vi "Write Test Result.vi"(9 "Position":u32, 10 "Test Passed":bool, 11 "Test Class.lvclass":refnum<class "Test Class.lvclass">) -> ()   [LabVIEW 2015]
uses:
  Classes/Application/Class/Application.lvclass
  Test Class.lvclass
  <vilib>/Cree, Inc/Cree Test Framework/Core Launcher/Core Launcher.lvlib
  <vilib>/Cree, Inc/Cree Test Framework/Core Launcher/Core Manager Methods -- Enum.ctl
  <vilib>/Cree, Inc/Cree Test Framework/Classes/Data/Data Repo/Class/Data Repo.lvclass
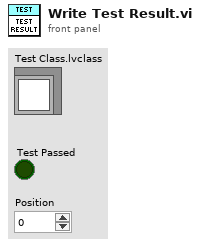
[diagram p1: front panel]
types:
  T1 = typedef "Core Launcher.lvlib/Core Manager Methods -- Enum.ctl" = enum16{"Spawn Objects", "Get Objects", "Destroy Objects"}
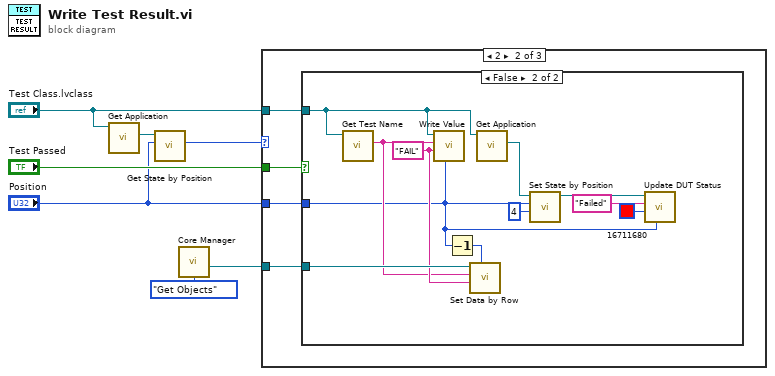
[diagram p0: block diagram]
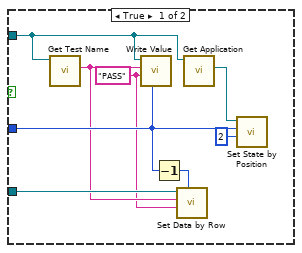
[diagram p3: hidden frame]
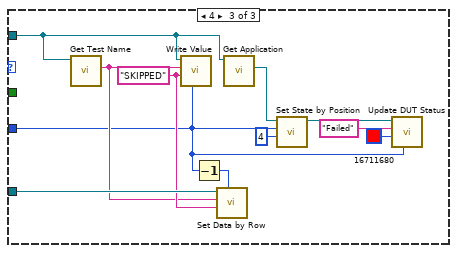
[diagram p4: hidden frame]
diagram:
  n1 = call "Get Application.vi"("Test Class in"="Test Class.lvclass") -> ("Application.lvlib:Application.lvclass"=w6:refnum<class "Application.lvclass">)  [unwired: 9 in, 1 out]
  n2 = call-dynamic "Get State by Position.vi"("Position"="Position", "Application in"=w6) -> ("State"=w4:u32)  [unwired: 7 in, 2 out]
  n3 = call <vilib>:"Core Manager.vi"("Method"=Core_Manager_Methods_--_Enum."Get Objects") -> ("Data Repo"=w2:refnum<class "Data Repo.lvclass">)  [unwired: 6 in, 4 out]
  n4 = case shown="2" w4 {
    tunnel: "Test Passed" -> [_ w11 _]
    tunnel: "Position" -> [_ w10 w31]
    tunnel: "Test Class.lvclass" -> [_ w9 w32]
    tunnel: w2 -> [_ w8 w41]
    frame Default {
    }
    frame 2 {
      n5 = case shown="False" w11 {
        tunnel: w10 -> [w16 w20]
        tunnel: w9 -> [w12 w21]
        tunnel: w8 -> [w17 w25]
        frame True {
          w13 = "PASS" ("Message")
          n6 = call "Get Test Name.vi"("Test Class in"=w12) -> ("Test Name"=w14:string)  [unwired: 9 in, 1 out]
          n7 = call "Write Value.vi"("Position"=w16, "Value"=w13, "Label"=w14, "Test Class in"=w12) -> ()  [unwired: 7 in, 1 out]
          n8 = Decrement(x=w16) -> (x-1=w15:u32)
          n9 = call <vilib>:"Set Data by Row.vi"("Row"=w15, "Value"=w13, "Header"=w14, "Acrobat Template in"=w17) -> ()  [unwired: 6 in, 2 out]
          n10 = call "Get Application.vi"("Test Class in"=w12) -> ("Application.lvlib:Application.lvclass"=w19:refnum<class "Application.lvclass">)  [unwired: 9 in, 1 out]
          n11 = call-dynamic "Set State by Position.vi"("State"=u32 2, "Position"=w16, "Application in"=w19) -> ()  [unwired: 7 in, 2 out]
        }
        frame False {
          w23 = "FAIL" ("Message")
          n12 = call "Get Test Name.vi"("Test Class in"=w21) -> ("Test Name"=w22:string)  [unwired: 9 in, 1 out]
          n13 = call "Write Value.vi"("Position"=w20, "Value"=w23, "Label"=w22, "Test Class in"=w21) -> ()  [unwired: 7 in, 1 out]
          n14 = Decrement(x=w20) -> (x-1=w24:u32)
          n15 = call <vilib>:"Set Data by Row.vi"("Row"=w24, "Value"=w23, "Header"=w22, "Acrobat Template in"=w25) -> ()  [unwired: 6 in, 2 out]
          n16 = call "Get Application.vi"("Test Class in"=w21) -> ("Application.lvlib:Application.lvclass"=w30:refnum<class "Application.lvclass">)  [unwired: 9 in, 1 out]
          n17 = call-dynamic "Set State by Position.vi"("State"=u32 4, "Position"=w20, "Application in"=w30) -> ("Application out"=w28:refnum<class "Application.lvclass">)  [unwired: 7 in, 1 out]
          n18 = call "Update DUT Status.vi"("Position"=w20, "BG Color"=u32 16711680, "Message ('')"="Failed", "Application in"=w28) -> ()  [unwired: 6 in, 2 out]
        }
      }
    }
    frame 4 {
      w34 = "SKIPPED" ("Message")
      n19 = call "Get Test Name.vi"("Test Class in"=w32) -> ("Test Name"=w33:string)  [unwired: 9 in, 1 out]
      n20 = call "Write Value.vi"("Position"=w31, "Value"=w34, "Label"=w33, "Test Class in"=w32) -> ()  [unwired: 7 in, 1 out]
      n21 = Decrement(x=w31) -> (x-1=w35:u32)
      n22 = call <vilib>:"Set Data by Row.vi"("Row"=w35, "Value"=w34, "Header"=w33, "Acrobat Template in"=w41) -> ()  [unwired: 6 in, 2 out]
      n23 = call "Get Application.vi"("Test Class in"=w32) -> ("Application.lvlib:Application.lvclass"=w40:refnum<class "Application.lvclass">)  [unwired: 9 in, 1 out]
      n24 = call-dynamic "Set State by Position.vi"("State"=u32 4, "Position"=w31, "Application in"=w40) -> ("Application out"=w38:refnum<class "Application.lvclass">)  [unwired: 7 in, 1 out]
      n25 = call "Update DUT Status.vi"("Position"=w31, "BG Color"=u32 16711680, "Message ('')"="Failed", "Application in"=w38) -> ()  [unwired: 6 in, 2 out]
    }
  }
